vi "S2C_Shared_Proc_Exit.vi"(8 "Error In":errorcluster) -> (0 "Error Out":errorcluster)   [LabVIEW 2024]
uses:
  S2C_Shared_Proc_Globals.vi
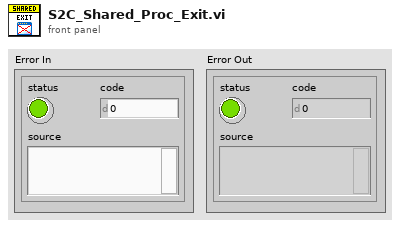
[diagram p1: front panel]
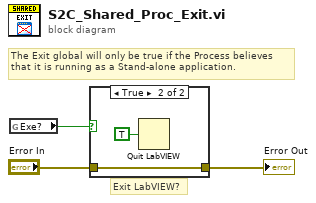
[diagram p0: block diagram]
diagram:
  # "The Exit global will only be true if the Process believes\nthat it is running as a Stand-alone application."
  # "Exit LabVIEW?"
  n1 = global read "S2C_Shared_Proc_Globals.vi" "Exe?"() -> (w1:bool)
  n2 = case shown="True" w1 {
    tunnel: "Error In" -> [w4 w5]
    tunnel: [w4 w5] -> w2
    frame False {
    }
    frame True {
      n3 = Quit LabVIEW(quit? (T)=TRUE) -> ()
    }
  }
  "Error Out" <- w2
